vi "Karol_Wrzesinski_praca_inzynierska.vi"() -> ()   [LabVIEW 2020]
uses:
  <vilib>/Instr/_visa.llb/VISA Configure Serial Port (Instr).vi
  <vilib>/Utility/file.llb/Write Delimited Spreadsheet (DBL).vi
panel:
  in  "stop":bool
  out "error out":errorcluster
  in  "sciezka zapisu":path
  in  "format (%.3f)":string="%.3f"
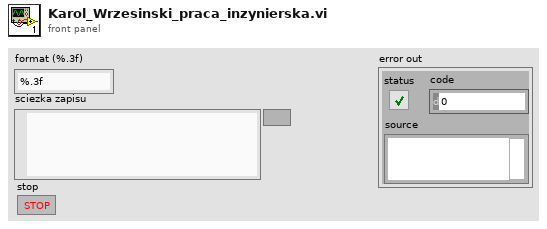
[diagram p1: front panel]
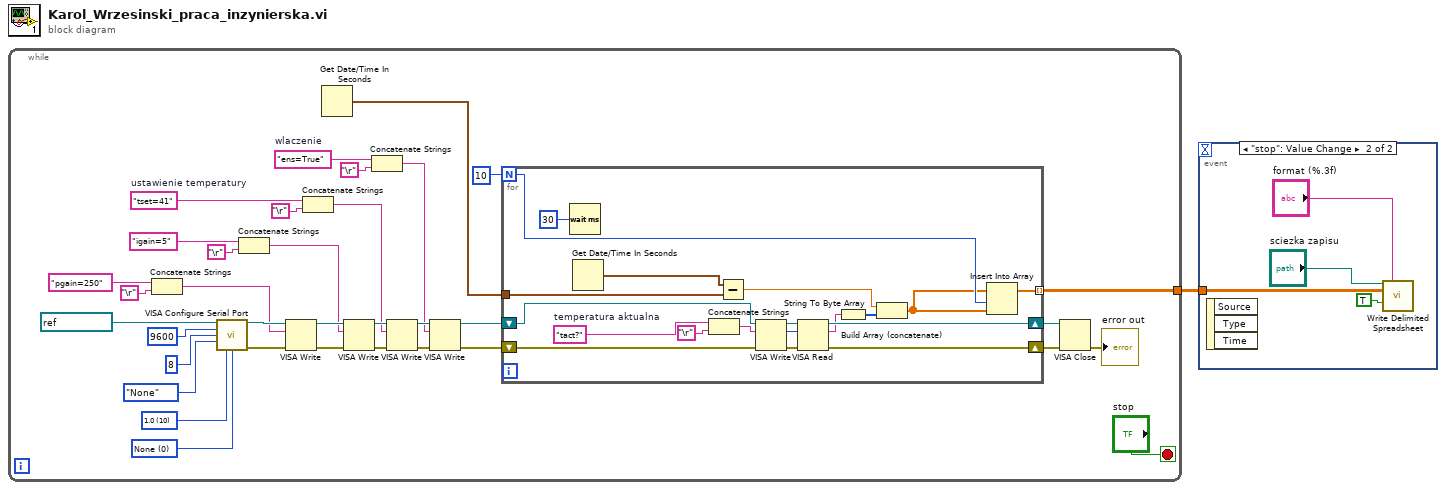
[diagram p0: block diagram]
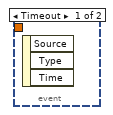
[diagram p2: hidden frame]
diagram:
  n1 = while {
    tunnel: [w2] -> w1
    stop <- "stop" stop-if-true
    w20 = "tset=41"  # ustawienie temperatury
    w18 = "ens=True"  # wlaczenie
    w11 = u16 0 items=["None", "XON/XOFF", "RTS/CTS", "XON/XOFF & RTS/CTS", "DTR/DSR", "XON/XOFF & DTR/DSR"] ("flow control (0:none)")
    w12 = u16 10 items=["1.0"=10, "1.5"=15, "2.0"=20] ("stop bits (10: 1 bit)")
    n2 = Concatenate Strings("pgain=250" ("string"), "\r") -> (w28:string)
    n3 = call-poly "VISA Configure Serial Port"("VISA resource name"=refnum<visa-resource-name> "COM1", "baud rate (9600)"=u32 9600, "data bits (8)"=u16 8, "parity (0:none)"=enum16{"None", "Odd", "Even", "Mark", "Space"}."None", "stop bits (10: 1 bit)"=w12, "flow control (0:none)"=w11) -> ("VISA resource name out"=w35:refnum<visa-resource-name>, "error out"=w34:errorcluster)  [unwired: 8 in]
    n4 = Concatenate Strings("igain=5" ("string"), "\r") -> (w29:string)
    n5 = VISA Write(VISA resource name=w35, write buffer=w28, error in (no error)=w34) -> (VISA resource name out=w31:refnum<visa-resource-name>, error out=w30:errorcluster)  [unwired: 1 out]
    n6 = Concatenate Strings(w20, "\r") -> (w25:string)
    n7 = Get Date/Time In Seconds() -> (seconds since 1Jan1904=w3:timestamp)
    n8 = VISA Write(VISA resource name=w31, write buffer=w29, error in (no error)=w30) -> (VISA resource name out=w33:refnum<visa-resource-name>, error out=w32:errorcluster)  [unwired: 1 out]
    n9 = Concatenate Strings(w18, "\r") -> (w10:string)
    n10 = VISA Write(VISA resource name=w33, write buffer=w25, error in (no error)=w32) -> (VISA resource name out=w27:refnum<visa-resource-name>, error out=w26:errorcluster)  [unwired: 1 out]
    n11 = VISA Write(VISA resource name=w27, write buffer=w10, error in (no error)=w26) -> (VISA resource name out=w7:refnum<visa-resource-name>, error out=w8:errorcluster)  [unwired: 1 out]
    n12 = for {
      N: 10 -> [w40]
      shift-right: [w53] -> w6
      shift-left: w8 -> [w55]
      shift-right: [w52] -> w5
      shift-left: w7 -> [w54]
      tunnel: w3 -> [w43]
      tunnel: [w39] -> w2 mode=indexing
      w47 = "tact?"  # temperatura aktualna
      n13 = Wait (ms)(milliseconds to wait=u32 30) -> ()  [unwired: 1 out]
      n14 = Get Date/Time In Seconds() -> (seconds since 1Jan1904=w44:timestamp)
      n15 = Concatenate Strings(w47, "\r") -> (w46:string)
      n16 = Subtract(x=w44, y=w43) -> (x-y=w38:dbl)
      n17 = VISA Write(VISA resource name=w54, write buffer=w46, error in (no error)=w55) -> (VISA resource name out=w48:refnum<visa-resource-name>, return count=w49:u32, error out=w50:errorcluster)
      n18 = VISA Read(VISA resource name=w48, byte count=w49, error in (no error)=w50) -> (VISA resource name out=w52:refnum<visa-resource-name>, read buffer=w41:string, error out=w53:errorcluster)  [unwired: 1 out]
      n19 = String To Byte Array(string=w41) -> (unsigned byte array=w42:u8[])
      n20 = Build Array (concatenate)(w38, w42) -> (w37:dbl[])
      n21 = Insert Into Array(array=w37, index=w40, new element=w37) -> (w39:dbl[])
    }
    n22 = VISA Close(VISA resource name=w5, error in (no error)=w6) -> (error out=→"error out":errorcluster)
  }
  n23 = event shown="[1] \"stop\": Value Change" {
    selector: _ -> [_ _]
    dyn-events: _ -> [_ _]
    timeout: _ -> [_ _]
    tunnel: w1 -> [_ w56]
    event Timeout {
      n24 = event-data() -> ()  [unwired: 1 in, 3 out]
    }
    event "stop": Value Change {
      n25 = event-data() -> ()  [unwired: 1 in, 3 out]
      n26 = call-poly <vilib>:"Write Delimited Spreadsheet.vi"("file path (dialog if empty)"="sciezka zapisu", "format (%.3f)"="format (%.3f)", "2D data"=w56, "append to file? (new file:F)"=TRUE) -> ()  [unwired: 10 in, 2 out]
    }
  }
